vi "readranges.vi"(11 "Range":dbl) -> (0 "error out":errorcluster, 2 "speed":dbl, 3 "angle":dbl)   [LabVIEW 2015]
uses:
  <vilib>/Utility/file.llb/Read Delimited Spreadsheet (DBL).vi
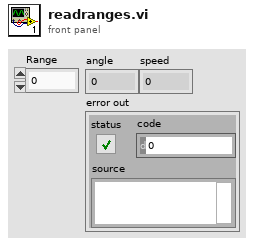
[diagram p1: front panel]
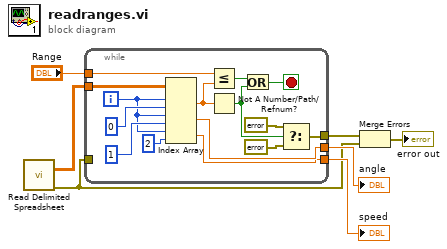
[diagram p0: block diagram]
diagram:
  n1 = call-poly <vilib>:"Read Delimited Spreadsheet.vi"() -> ("all rows"=w4:dbl[][], "error out"=w3:errorcluster)  [unwired: 10 in, 4 out]
  n2 = while {
    tunnel: "Range" -> [w15]
    tunnel: [w19] -> w6
    tunnel: [w18] -> w5
    tunnel: w4 -> [w17]
    tunnel: w3 -> [_]
    tunnel: [w9] -> w2
    i -> [w16]
    stop <- w12 stop-if-true
    n3 = Index Array(array=w17, index (row) #1=w16, index (col) #1=0 ("disabled index (col)"), index (row) #2=w16, index (col) #2=1 ("disabled index (col)"), index (row) #3=w16, index (col) #3=2 ("disabled index (col)")) -> (element #1=w14:dbl, element #2=w19:dbl, element #3=w18:dbl)
    n4 = Less Or Equal?(x=w15, y=w14) -> (x <= y?=w13:bool)
    n5 = Not A Number/Path/Refnum?(number/path/refnum=w14) -> (NaN/Path/Refnum?=w10:bool)
    n6 = Or(x=w13, y=w10) -> (x .or. y?=w12:bool)
    n7 = Select(t=errorcluster {"status"=TRUE, "code"=9001, "source"="Out of range!"} ("error constant"), s=w10, f=errorcluster {"status"=FALSE, "code"=0, "source"=""}) -> (s? t:f=w9:errorcluster)
  }
  "speed" <- w5
  "angle" <- w6
  n8 = Merge Errors(w2, w3) -> (→"error out":errorcluster)
